vi "Qn_X.vi"(8 "Type":string, 11 "shape":string) -> (3 "Qn":dbl[](array[numeric]))   [LabVIEW 2015]
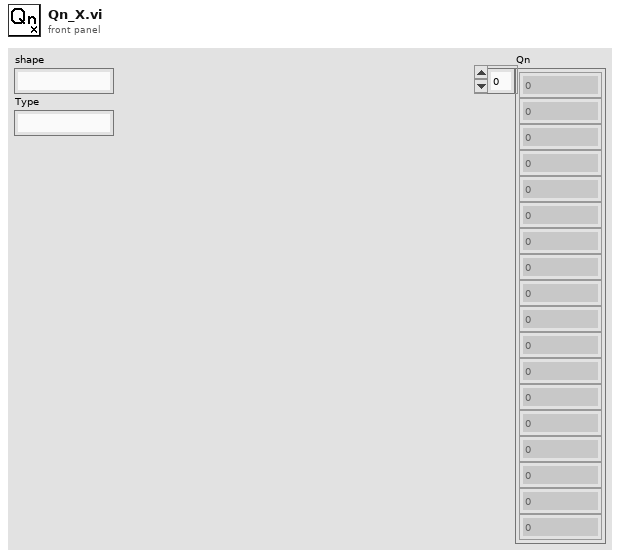
[diagram p1: front panel]
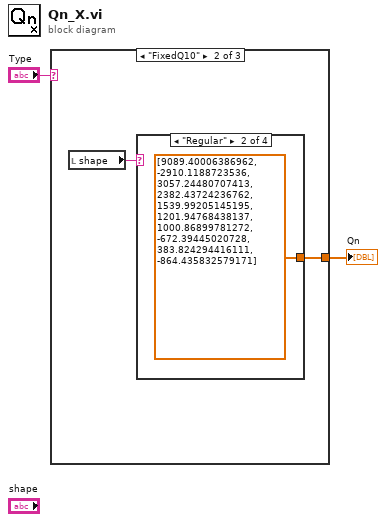
[diagram p0: block diagram]
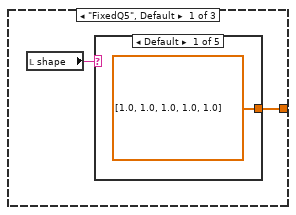
[diagram p2: hidden frame]
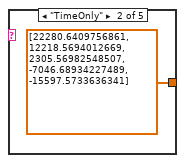
[diagram p3: hidden frame]
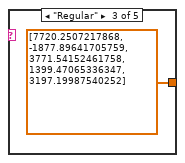
[diagram p4: hidden frame]
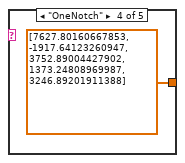
[diagram p5: hidden frame]
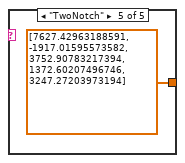
[diagram p6: hidden frame]
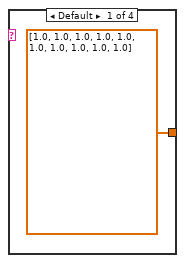
[diagram p7: hidden frame]
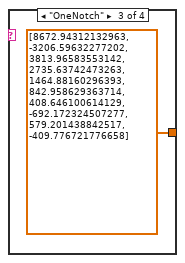
[diagram p8: hidden frame]
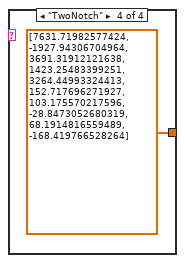
[diagram p9: hidden frame]
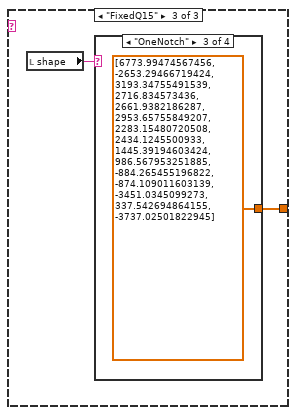
[diagram p10: hidden frame]
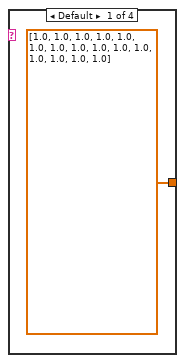
[diagram p11: hidden frame]
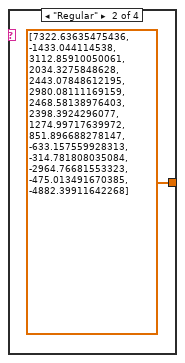
[diagram p12: hidden frame]
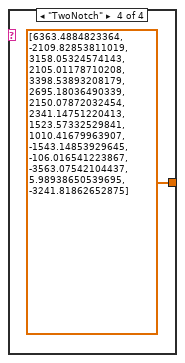
[diagram p13: hidden frame]
diagram:
  n1 = case shown="\"FixedQ10\"" "Type" {
    tunnel: [w4 w10 w16] -> w2
    frame "FixedQ5", Default {
      n2 = local read "shape"() -> (w3:string)
      n3 = case shown="Default" w3 {
        tunnel: [dbl[] [1.0, 1.0, 1.0, 1.0, 1.0] ("Qn") dbl[] [22280.6409756861, 12218.5694012669, 2305.56982548507, -7046.68934227489, -15597.5733636341] ("Qn") dbl[] [7720.2507217868, -1877.89641705759, 3771.54152461758, 1399.47065336347, 3197.19987540252] ("Qn") dbl[] [7627.80160667853, -1917.64123260947, 3752.89004427902, 1373.24808969987, 3246.89201911388] ("Qn") dbl[] [7627.42963188591, -1917.01595573582, 3752.90783217394, 1372.60207496746, 3247.27203973194] ("Qn")] -> w4
        frame Default {
        }
        frame "TimeOnly" {
        }
        frame "Regular" {
        }
        frame "OneNotch" {
        }
        frame "TwoNotch" {
        }
      }
    }
    frame "FixedQ10" {
      n4 = local read "shape"() -> (w11:string)
      n5 = case shown="\"Regular\"" w11 {
        tunnel: [dbl[] [1.0, 1.0, 1.0, 1.0, 1.0, 1.0, 1.0, 1.0, 1.0, 1.0] ("Qn") dbl[] [9089.40006386962, -2910.1188723536, 3057.24480707413, 2382.43724236762, 1539.99205145195, 1201.94768438137, 1000.86899781272, -672.39445020728, 383.824294416111, -864.435832579171] ("Qn") dbl[] [8672.94312132963, -3206.59632277202, 3813.96583553142, 2735.63742473263, 1464.88160296393, 842.958629363714, 408.646100614129, -692.172324507277, 579.201438842517, -409.776721776658] ("Qn") dbl[] [7631.71982577424, -1927.94306704964, 3691.31912121638, 1423.25483399251, 3264.44993324413, 152.717696271927, 103.175570217596, -28.8473052680319, 68.1914816559489, -168.419766528264] ("Qn")] -> w10
        frame Default {
        }
        frame "Regular" {
        }
        frame "OneNotch" {
        }
        frame "TwoNotch" {
        }
      }
    }
    frame "FixedQ15" {
      n6 = local read "shape"() -> (w17:string)
      n7 = case shown="\"OneNotch\"" w17 {
        tunnel: [dbl[] [1.0, 1.0, 1.0, 1.0, 1.0, 1.0, 1.0, 1.0, 1.0, 1.0, 1.0, 1.0, 1.0, 1.0, 1.0] ("Qn") dbl[] [7322.63635475436, -1433.044114538, 3112.85910050061, 2034.3275848628, 2443.07848612195, 2980.08111169159, 2468.58138976403, 2398.3924296077, 1274.99717639972, 851.896688278147, -633.157559928313, -314.781808035084, -2964.76681553323, -475.013491670385, -4882.39911642268] ("Qn") dbl[] [6773.99474567456, -2653.29466719424, 3193.34755491539, 2716.834573436, 2661.9382186287, 2953.65755849207, 2283.15480720508, 2434.1245500933, 1445.39194603424, 986.567953251885, -884.265455196822, -874.109011603139, -3451.0345099273, 337.542694864155, -3737.02501822945] ("Qn") dbl[] [6363.4884823364, -2109.82853811019, 3158.05324574143, 2105.01178710208, 3398.53893208179, 2695.18036490339, 2150.07872032454, 2341.14751220413, 1523.57332529841, 1010.41679963907, -1543.14853929645, -106.016541223867, -3563.07542104437, 5.98938650539695, -3241.81862652875] ("Qn")] -> w16
        frame Default {
        }
        frame "Regular" {
        }
        frame "OneNotch" {
        }
        frame "TwoNotch" {
        }
      }
    }
  }
  "Qn" <- w2
